vi "test_Add Single Ch. Comparison .vi"(8 "error in (no error)":errorcluster, 11 "TestCase in":refnum<class "Instrument Addon Scripting API Channels Unit Tests.lvclass">) -> (0 "error out":errorcluster, 3 "TestCase out":refnum<class "Instrument Addon Scripting API Channels Unit Tests.lvclass">)   [LabVIEW 2018, in "Instrument Addon Scripting API Channels Unit Tests.lvclass"]
uses:
  Instrument Addon Scripting API Channels Unit Tests.lvclass
  APIs/Scripting API/TypeDefs/Single Channel Comparison Settings.ctl
  Addon/Addon Shared/SubVIs/Constants.vi
  <vilib>/NI/NI VeriStand Advanced SysDef API/_SubVIs/SysDef.Search.GUID.vi
  APIs/Scripting API/Channels/Create Data Channel - Single Channel - Comparison.vi
  <vilib>/NI Veristand/Custom Device API/Get Item Property (String).vi
  <vilib>/NI/NI VeriStand Advanced SysDef API/_SubVIs/SysDef.Search.GUIDs.vi
  <vilib>/addons/_JKI Toolkits/VI Tester/TestCase.llb/TestCase.lvclass
  Instrument Addon Scripting API Test Assets/Instrument Addon Scripting API Test Assets.lvclass
  <vilib>/NI/NI VeriStand Advanced SysDef API/SysDef API/Advanced System Definition.lvlib
  Addon/Addon Shared/Instrument Addon Shared.lvlib
  <vilib>/NI Veristand/Custom Device API/Custom Device API.lvlib
  APIs/Scripting API/Instrument Addon Scripting API.lvlib
  C:/Program Files (x86)/National Instruments/LabVIEW 2018/vi.lib/addons/_JKI Toolkits/VI Tester/TestCase.llb/TestCase.lvclass
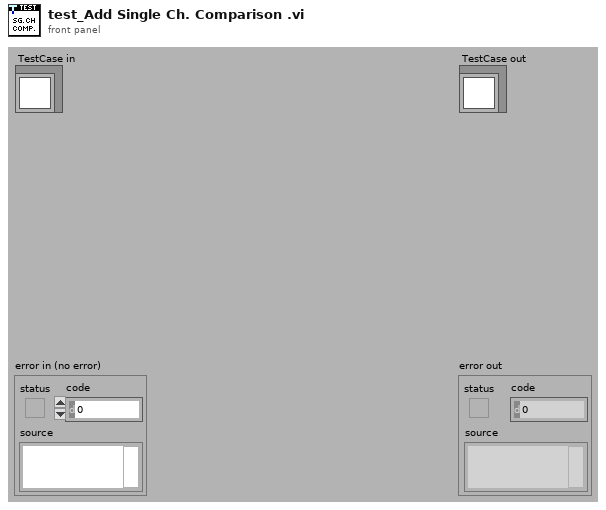
[diagram p1: front panel]
types:
  T1 = typedef "Instrument Addon Scripting API.lvlib/Single Channel Comparison Settings.ctl" = cluster{"Expected String(case sensitive)":string, "Default Value":dbl, "Units":string}
  T2 = typedef "Custom Device API.lvlib/Custom Device Item Ref.ctl" = u64
  T3 = typedef "Custom Device API.lvlib/Custom Device Channel.ctl" = cluster{"Type":T4, "Units":string, "Default Value":dbl, "Faultable":bool, "Scalable":bool}
  T4 = typedef "Custom Device API.lvlib/Custom Device Channel Type.ctl" = enum16{"Input", "Output"}
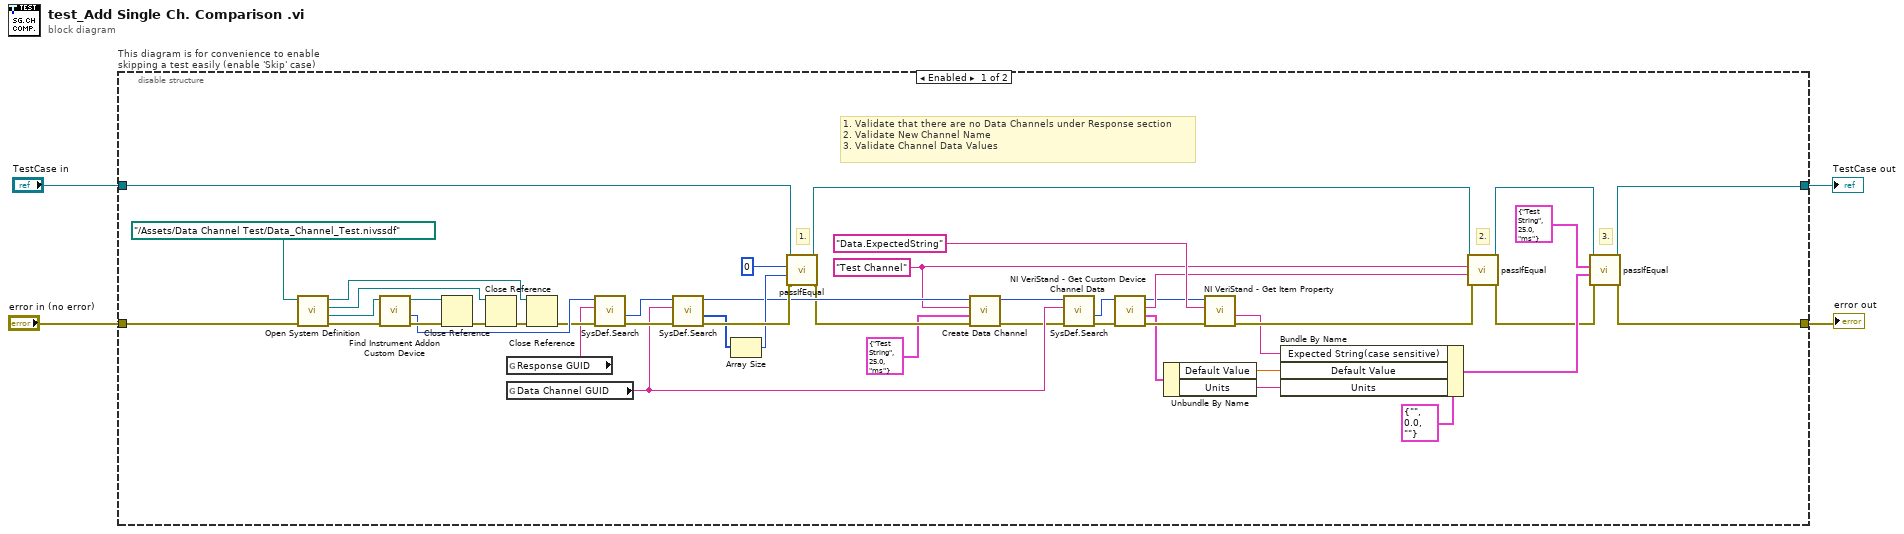
[diagram p0: block diagram]
diagram:
  n1 = disable-structure "This diagram is for convenience to enable skipping a test easily (enable 'Skip' case)" shown="Enabled" {
    disable-tunnel: "TestCase in" -> [w22 w54]
    disable-tunnel: [w50 w52] -> w1
    disable-tunnel: [w49 w53] -> w3
    disable-tunnel: "error in (no error)" -> [w39 w51]
    frame Enabled {
      w15 = "Test Channel" ("Name")
      # "3."
      # "2."
      # "1. Validate that there are no Data Channels under Response section\n2. Validate New Channel Name\n3. Validate Channel Data Values"
      # "1."
      n2 = call "Open System Definition.vi"("error in (no error)"=w39, "System Definition File"=path "../Assets/Data Channel Test/Data_Channel_Test.nivssdf") -> ("error out"=w48:errorcluster, "Target Refnum"=w47:refnum<k24>, "Root Refnum"=w43:refnum<k24>, "System Definition Refnum"=w44:refnum<k24>)  [unwired: 6 in]
      n3 = call "Find Instrument Addon Custom Device.vi"("error in"=w48, "target in"=w47) -> ("error out"=w40:errorcluster, "NodeID"=w38:u64, "target out"=w41:refnum<k24>)  [unwired: 7 in]
      n4 = Close Reference(reference=w41, error in (no error)=w40) -> (error out=w42:errorcluster)
      n5 = Close Reference(reference=w43, error in (no error)=w42) -> (error out=w45:errorcluster)
      n6 = global read "Constants.vi" "Response GUID"() -> (w36:string)
      n7 = global read "Constants.vi" "Data Channel GUID"() -> (w33:string)
      n8 = Close Reference(reference=w44, error in (no error)=w45) -> (error out=w37:errorcluster)
      n9 = call-poly <vilib>:"SysDef.Search.vi"("error in (no error)"=w37, "GUID"=w36, "nodeID"=w38) -> ("error out"=w34:errorcluster, "Value out"=w35:u64)  [unwired: 5 in, 2 out]
      n10 = call-poly <vilib>:"SysDef.Search.vi"("error in (no error)"=w34, "GUID"=w33, "nodeID"=w35) -> ("error out"=w20:errorcluster, "Values Out"=w19:u64[], "nodeID out"=w16:u64)  [unwired: 5 in, 1 out]
      n11 = Array Size(array=w19) -> (size(s)=w18:i32)
      n12 = call-dynamic "passIfEqual.vi"("error in (no error)"=w20, "y"=w18, "x"=0 ("size(s)"), "TestCase in"=w22) -> ("error out"=w14:errorcluster, "TestCase out"=w21:refnum<class "Instrument Addon Scripting API Channels Unit Tests.lvclass">)  [unwired: 6 in]
      n13 = call-poly "Create Data Channel.vi"("Error In"=w14, "Settings"=T1 {"Expected String(case sensitive)"="Test String", "Default Value"=25.0, "Units"="ms"}, "Name"=w15, "Message Refnum In"=w16) -> ("Error Out"=w12:errorcluster, "Message Refnum Out"=w13:T2)  [unwired: 5 in, 1 out]
      n14 = call-poly <vilib>:"SysDef.Search.vi"("error in (no error)"=w12, "GUID"=w33, "nodeID"=w13) -> ("error out"=w32:errorcluster, "Value out"=w9:u64)  [unwired: 5 in, 2 out]
      n15 = call <vilib>:"NI VeriStand - Get Custom Device Channel Data.vi"("error in (no error)"=w32, "Channel Ref in"=w9) -> ("error out"=w31:errorcluster, "Channel"=w30:T3, "Channel Name"=w25:string, "Channel Ref out"=w11:T2)  [unwired: 4 in, 2 out]
      n16 = Unbundle By Name(w30) -> ("Default Value"=w29:dbl, "Units"=w28:string)
      n17 = call-poly <vilib>:"NI VeriStand - Get Item Property.vi"("error in (no error)"=w31, "Property Name"="Data.ExpectedString", "Item Ref in"=w11) -> ("error out"=w10:errorcluster, "Value"=w6:string)  [unwired: 5 in, 2 out]
      n18 = Bundle By Name(cluster=T1 {"Expected String(case sensitive)"="", "Default Value"=0.0, "Units"=""} ("Settings"), "Expected String(case sensitive)"=w6, "Default Value"=w29, "Units"=w28) -> (w24:T1)
      n19 = call-dynamic "passIfEqual.vi"("error in (no error)"=w10, "y"=w25, "x"=w15, "TestCase in"=w21) -> ("error out"=w23:errorcluster, "TestCase out"=w26:refnum<class "Instrument Addon Scripting API Channels Unit Tests.lvclass">)  [unwired: 6 in]
      n20 = call-dynamic "passIfEqual.vi"("error in (no error)"=w23, "y"=w24, "x"=T1 {"Expected String(case sensitive)"="Test String", "Default Value"=25.0, "Units"="ms"} ("Settings"), "TestCase in"=w26) -> ("error out"=w49:errorcluster, "TestCase out"=w50:refnum<class "Instrument Addon Scripting API Channels Unit Tests.lvclass">)  [unwired: 6 in]
    }
    frame Disabled {
      # "skip test result while test is under development"
      n21 = call <vilib>:"skip.vi"("error in (no error)"=w51, "TestCase in"=w54) -> ("error out"=w53:errorcluster, "TestCase out"=w52:refnum<class "Instrument Addon Scripting API Channels Unit Tests.lvclass">)  [unwired: 8 in]
    }
  }
  "error out" <- w3
  "TestCase out" <- w1
